vi "ConstantRateHistUnshaken.vi"() -> ()   [LabVIEW 2015]
uses:
  <vilib>/Utility/file.llb/Read Delimited Spreadsheet (DBL).vi
panel:
  in  "Unshaken Water":path=path "C:/Users/Brian/Desktop/New folder/week8/Unshaken_Water"
  out "Waveform Graph 2":dynamicdata(graph)=[{"t0"=timestamp(1 s since 1904-01-01), "dt"=2.0, "Y"=[1.9660320397143503e-24, 1.283579840942134e-21, 2.622822759322242e-19, 2.5681793846031902e-17, 1.4699870339341842e-15, 5.5126212206855714e-14, 1.4584631611991872e-12, 2.867298403178021e-11, 4.352993034819423e-10, 5.256607688666258e-09, 5.169429726812739e-08, 4.2199763245248233e-07, 2.9053645146368968e-06, 1.709716184357092e-05, 8.698478358640886e-05, 0.00038640928873993137, 0.0015117522224159055, 0.005248542465180647, 0.01627969729868915, 0.045385349959381996, 0.11433897652094524, 0.2615792105434118, 0.5458437649439452, 1.0431485694385139, 1.8325049038505374, 2.969229221797762, 4.451490589299628, 6.192869158891884, 8.016294400288425, 9.679208720603325, 10.927136863844991, 11.559073725214317, 11.48100092886219, 10.727835811053605, 9.447266839998486, 7.854214237675692, 6.174490773082787, 4.596874708945658, 3.2457385990807603, 2.17644487445035, 1.3878070164268121, 0.8425469139519608, 0.4875883778217309, 0.26927347674700197, 0.14206244187524864, 0.07167276530076044, 0.03461326414461049, 0.01601587348446922, 0.007106692621847243, 0.0030266795919425193], "attributes"=variant("NI_ChannelName"=variant(string " (Best fit)"), "NI_ExpIsRelativeTime"=variant(bool TRUE), "NI_ExpStartTimeStamp"=variant(timestamp timestamp(3531847333.377577 s since 1904-01-01)), "NI_ExpTimeStamp"=variant(timestamp timestamp(3531847333.377577 s since 1904-01-01)), "NI_ExpXDimension"=variant(string "BIN"), "NI_OriginalChannelName"=variant(string ""))}, {"t0"=timestamp(1 s since 1904-01-01), "dt"=2.0, "Y"=[0.0, 0.0, 0.0, 0.0, 0.0, 0.0, 0.0, 0.0, 0.0, 0.0, 0.0, 0.0, 0.0, 0.0, 0.0, 0.0, 0.0, 0.0, 0.0, 0.0, 0.0, 0.0, 0.0, 1.0, 3.0, 1.0, 7.0, 3.0, 13.0, 6.0, 13.0, 9.0, 12.0, 9.0, 17.0, 2.0, 6.0, 2.0, 9.0, 1.0, 1.0, 1.0, 0.0, 0.0, 0.0, 0.0, 0.0, 0.0, 0.0, 0.0], "attributes"=variant("NI_ChannelName"=variant(string " (Histogram)"), "NI_ExpIsRelativeTime"=variant(bool TRUE), "NI_ExpStartTimeStamp"=variant(timestamp timestamp(3531847333.377577 s since 1904-01-01)), "NI_ExpTimeStamp"=variant(timestamp timestamp(3531847333.377577 s since 1904-01-01)), "NI_ExpXDimension"=variant(string "BIN"), "NI_OriginalChannelName"=variant(string ""))}]
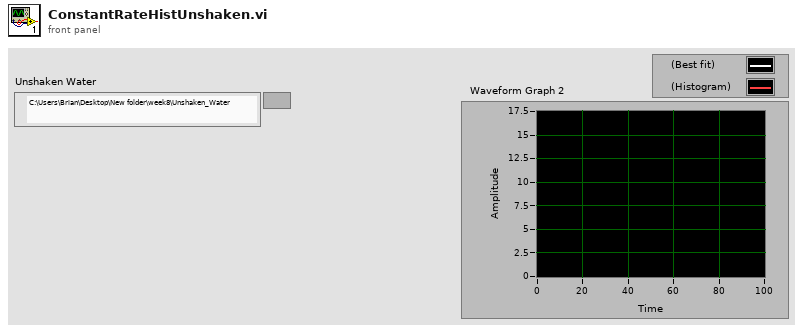
[diagram p1: front panel]
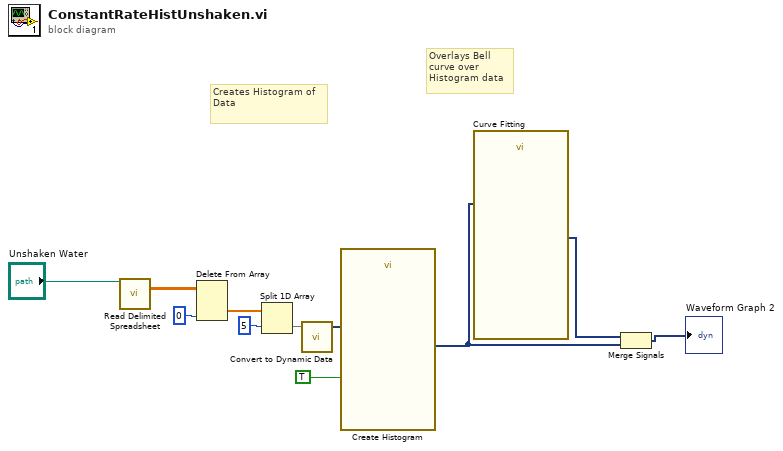
[diagram p0: block diagram]
diagram:
  # "Overlays Bell curve over Histogram data"
  # "Creates Histogram of Data"
  n1 = call-poly <vilib>:"Read Delimited Spreadsheet.vi"("file path (dialog if empty)"="Unshaken Water") -> ("all rows"=w3:dbl[][])  [unwired: 9 in, 5 out]
  n2 = Delete From Array(array=w3, index (col)=0) -> (deleted portion=w5:dbl[])  [unwired: 2 in, 1 out]
  n3 = Split 1D Array(array=w5, index=5) -> (second subarray=w11:dbl[])  [unwired: 1 out]
  n4 = call "Convert to Dynamic Data"("Array"=w11) -> ("Dynamic Data Type"=w1:dynamicdata)  [unwired: 3 in]
  n5 = call "Create Histogram"("Enable"=TRUE, "Signal"=w1) -> ("Histogram"=w8:dynamicdata)  [unwired: 8 in, 1 out]
  n6 = call "Curve Fitting"("Signals"=w8) -> ("best fit"=w7:dynamicdata)  [unwired: 6 in, 4 out]
  n7 = Merge Signals(w7, w8) -> (→"Waveform Graph 2":dynamicdata)
